vi "data_load_display_trend_fft_mea_coll_v4.vi"() -> ()   [LabVIEW 2020]
uses:
  <vilib>/Analysis/2dsp.llb/Real FFT.vi
  <vilib>/Utility/file.llb/Read Delimited Spreadsheet (DBL).vi
  <vilib>/Utility/file.llb/Read Delimited Spreadsheet (string).vi
  <vilib>/Analysis/NI_AALPro.lvlib
  <vilib>/rvi/Analysis/host/Public/NI_FpgaMspHost.lvlib
  <vilib>/ptbypt/NI_PtbyPt.lvlib
panel:
  out "x-y":dbl
  out "XY Graph 2":T1(graph)
  out "Waveform Graph":dbl[][](graph)
  out "XY Graph":cluster{dbl[], dbl[]}(graph)
  out "magnitude 2":dbl[](array[numeric])
  out "phase 2":dbl[](array[numeric])
  out "signal from each selected frequency":dbl[][](array[numeric])
  out "ploted signal from each selected frequency":dbl[][](graph)
  out "plot restored signal":dbl[](graph)
  out "restored signal":dbl[](array[numeric])
  out "phase":dbl format="%0.2f"
  out "magnitude":dbl format="%0.2f"
  out "magnitude plot":dbl[](graph)
  out "phase plot":dbl[](graph)
  out "magnitudes":dbl[](array[numeric])
  out "phasees":dbl[](array[numeric])
  out "df (Hz)":dbl
  out "size(s)":i32
  out "xf (frequency)":dbl[](array[numeric])
  in  "decimating factor":i32=3
  out "xf (sample Vs frequency )":dbl[][](array[numeric]) format="%#20_5g"
  out "Imaginary values":dbl[](array[numeric])
  out "real  values":dbl[](array[numeric])
  out "real plot":dbl[](graph)
  out "imaginary plot":dbl[](graph)
  out "Time Domain sequence":cluster{i32, dbl, dbl[]}(graph)
  out "Frequency Interval: delta(f)":dbl
  out "Spectrum plot":cluster{i32, dbl, "spectrum out":dbl[]}(graph)
  out "Remove trend":cluster{"all rows":dbl[], dbl[]}(graph)
  out "Time vs Acceleration  find trend graph":T2(graph)
  out "array w/ subset deleted":dbl[][](array[numeric])
  out "first row":string[][](array[string])
  out "time":dbl[](array[numeric])
  out "Acceleration":dbl[](array[numeric])
  out "Time vs Acceleration graph":cluster{"all rows":dbl[], "all rows":dbl[]}(graph)
  out "stripped path":path
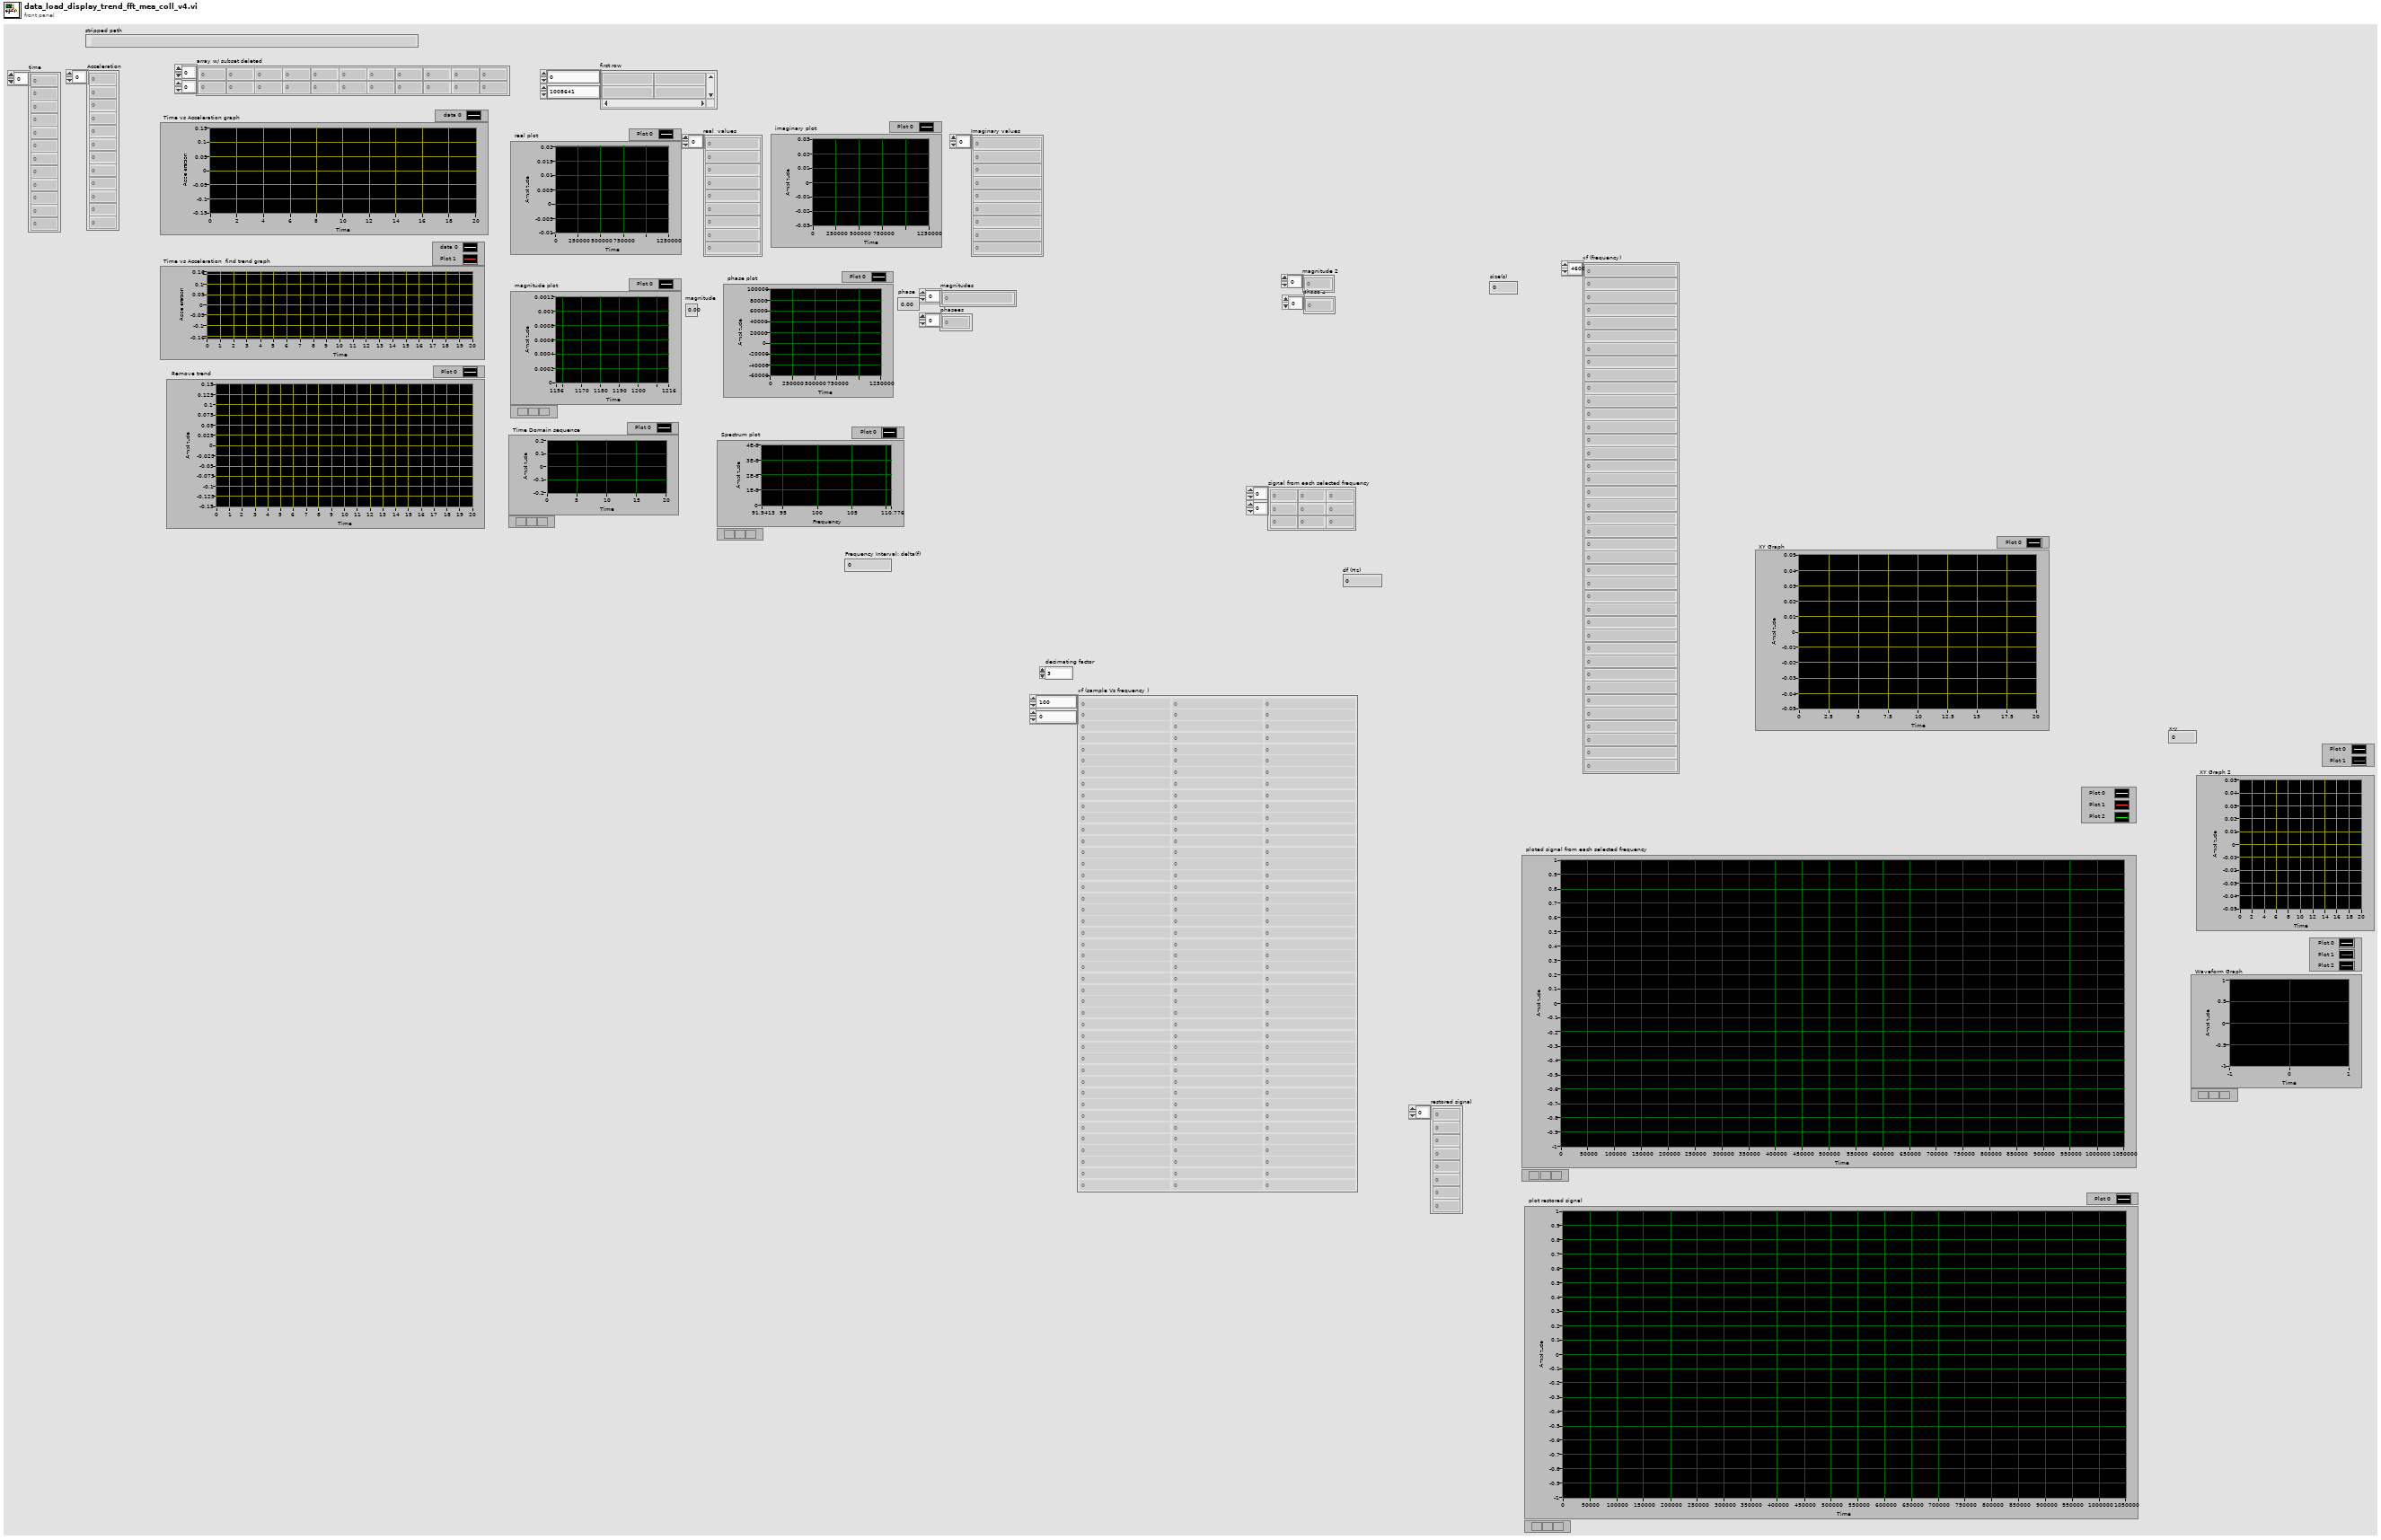
[diagram p1: front panel]
types:
  T1 = cluster{"all rows":dbl[], "Best Linear Fit":dbl[]}[]
  T2 = cluster{"all rows":dbl[], "Best Linear Fit":dbl[]}
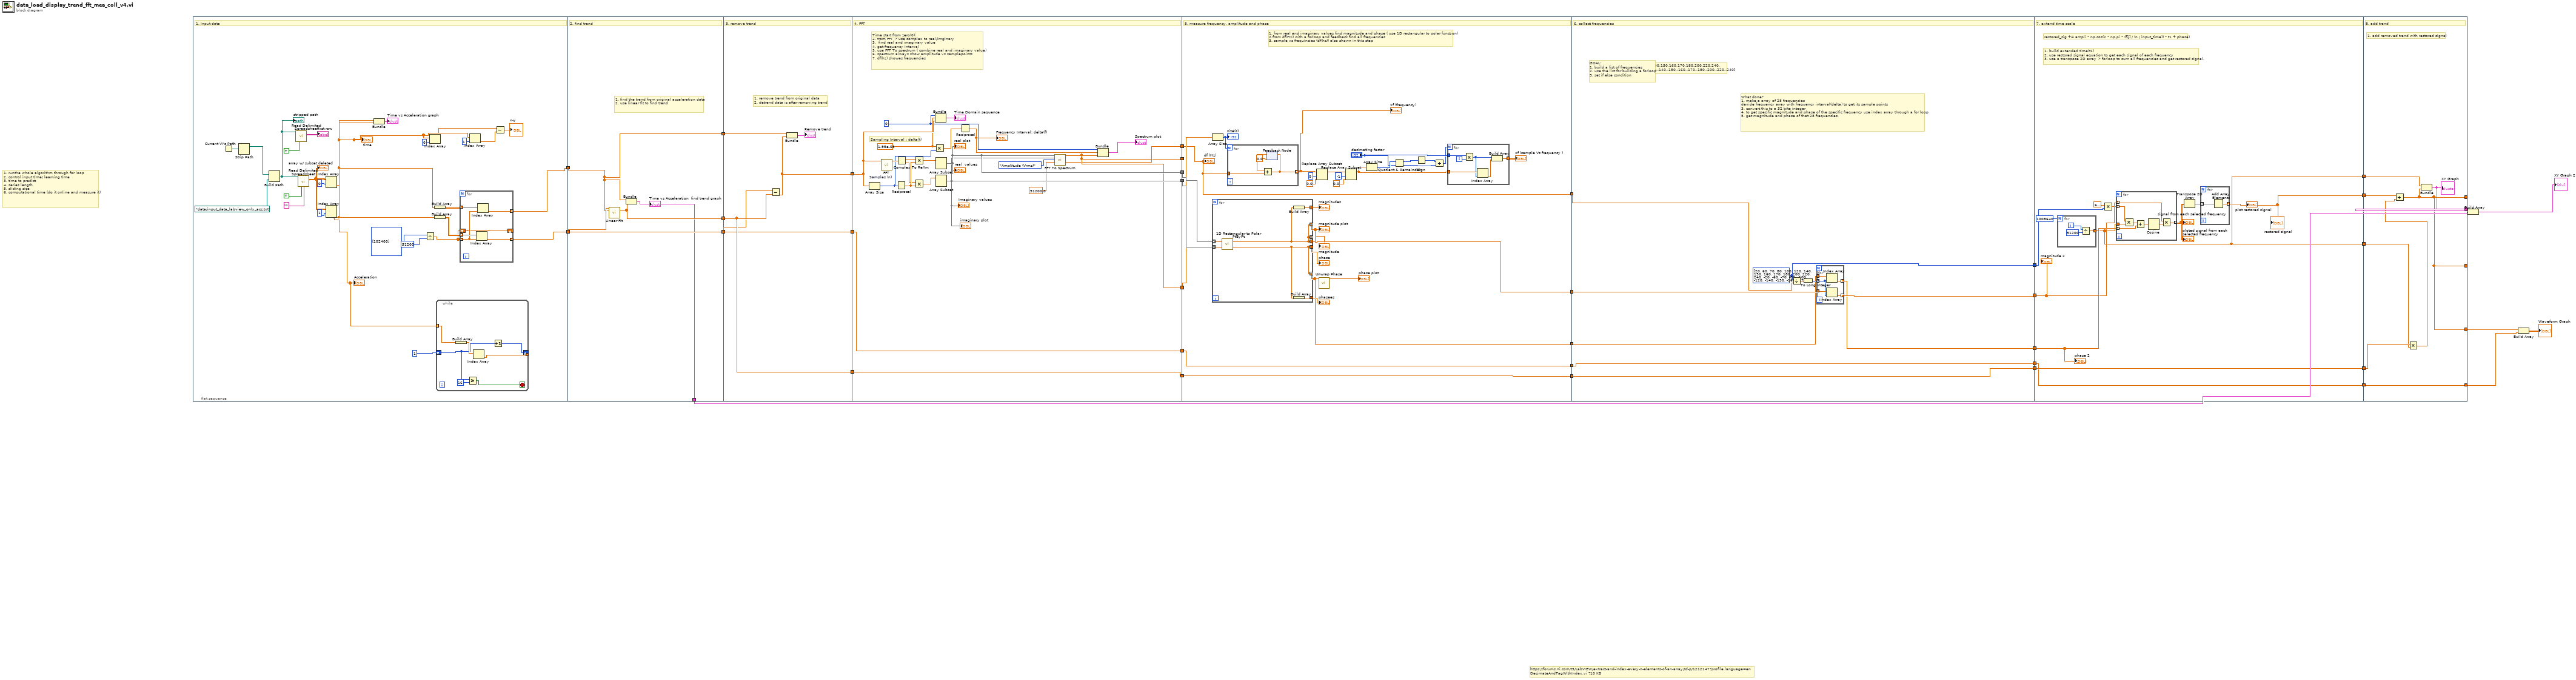
[diagram p0: block diagram]
diagram:
  # "1. runthe whole algorithm through for loop \n2. control input time/ learning time\n3. time to predict\n4. series length\n5. sliding size\n6. computational time (do it online and measure it)"
  # "https://forums.ni.com/t5/LabVIEW/extract-and-index-every-n-elements-of-an-array/td-p/1212147?profile.language=en\nDecimateAndTagWithIndex.vi ?10 KB"
  n1 = flat-sequence {
    tunnel: [w44] -> w36
    tunnel: [w45] -> w35
    tunnel: w36 -> [w79]
    tunnel: [w80] -> w34
    tunnel: [w79] -> w33
    tunnel: [w78] -> w32
    tunnel: w35 -> [w78]
    tunnel: [w77] -> w2
    tunnel: w34 -> [w82]
    tunnel: w33 -> [w81]
    tunnel: w32 -> [w85]
    tunnel: [w84] -> w31
    tunnel: [w82] -> w30
    tunnel: [w81] -> w29
    tunnel: w31 -> [w101]
    tunnel: [w98] -> w28
    tunnel: [w97] -> w27
    tunnel: [w89] -> w26
    tunnel: [w90] -> w25
    tunnel: [w89] -> w24
    tunnel: [w87] -> w23
    tunnel: w30 -> [w87]
    tunnel: w29 -> [w86]
    tunnel: [w86] -> w22
    tunnel: w28 -> [w135]
    tunnel: w27 -> [w134]
    tunnel: w26 -> [_]
    tunnel: w25 -> [w113]
    tunnel: w24 -> [w128]
    tunnel: [w113] -> w21
    tunnel: [w112] -> w20
    tunnel: [w110] -> w19
    tunnel: [w109] -> w18
    tunnel: w23 -> [w109]
    tunnel: w22 -> [w108]
    tunnel: [w108] -> w17
    tunnel: w21 -> [w161]
    tunnel: [w158] -> w16
    tunnel: w20 -> [w157]
    tunnel: w19 -> [w156]
    tunnel: [w155] -> w15
    tunnel: [w154] -> w14
    tunnel: [w153] -> w13
    tunnel: w18 -> [w153]
    tunnel: w17 -> [w152]
    tunnel: [w152] -> w12
    tunnel: w16 -> [w176]
    tunnel: w15 -> [w177]
    tunnel: w14 -> [w172]
    tunnel: [w170] -> w11
    tunnel: [w169] -> w10
    tunnel: w13 -> [w169]
    tunnel: [w168] -> w9
    tunnel: [w168] -> w8
    tunnel: w12 -> [w167]
    tunnel: [w167] -> w7
    tunnel: w11 -> [w199]
    tunnel: w10 -> [w197]
    tunnel: w9 -> [w198]
    tunnel: w8 -> [w196]
    tunnel: [w193] -> _
    tunnel: [w194] -> w5
    tunnel: w7 -> [w194]
    tunnel: [w193] -> _
    tunnel: [w193] -> w6
    tunnel: [w192] -> w3
    frame #0 {
      # "1. Input data"
      n2 = Current VI's Path() -> (path=w55:path)
      n3 = Strip Path(path=w55) -> (stripped path=w54:path)  [unwired: 1 out]
      n4 = Build Path(base path=w54, name or relative path=path "data/input_data_labview_only_acc.txt") -> (appended path=w52:path)
      "stripped path" <- w52
      n5 = call-poly <vilib>:"Read Delimited Spreadsheet.vi"("file path (dialog if empty)"=w52, "transpose? (F)"=TRUE) -> ("all rows"=→"first row":string[][])  [unwired: 8 in, 5 out]
      n6 = call-poly <vilib>:"Read Delimited Spreadsheet.vi"("file path (dialog if empty)"=w52, "transpose? (F)"=TRUE, "delimiter (\\t)"="" ("delimiter (\\t)")) -> ("all rows"=w57:dbl[][])  [unwired: 7 in, 5 out]
      "array w/ subset deleted" <- w57
      n7 = Index Array(array=w57, index (row)=0) -> (element=w42:dbl[])  [unwired: 1 in]
      "time" <- w42
      n8 = Index Array(array=w57, index (row)=1) -> (element=w49:dbl[])  [unwired: 1 in]
      "Acceleration" <- w49
      n9 = Bundle("all rows"=w42, "all rows"=w49) -> (→"Time vs Acceleration graph":cluster{"all rows":dbl[], "all rows":dbl[]})  [unwired: 1 in]
      n10 = Divide(x=i32[] [102400], y=51200) -> (x/y=w43:dbl[])
      n11 = Index Array(array=w42, index=0) -> (element=w39:dbl)
      n12 = Build Array(w42) -> (w50:dbl[][])
      n13 = Build Array(w49) -> (w48:dbl[][])
      n14 = while {
        tunnel: w49 -> [w76] mode=indexing
        tunnel: [w74] -> _ mode=indexing
        shift-right: [w73] -> _
        shift-left: 1 ("index (row)") -> [w72]
        stop <- w70 stop-if-true
        n15 = Build Array(w76) -> (w75:dbl[])
        n16 = Greater Or Equal?(x=w72, y=16) -> (x >= y?=w70:bool)
        n17 = Index Array(array=w75) -> (element=w74:dbl)  [unwired: 1 in]
        n18 = Increment(x=w72) -> (x+1=w73:i32)
      }
      n19 = for {
        tunnel: w50 -> [w69] mode=indexing
        tunnel: w48 -> [w68] mode=indexing
        tunnel: w43 -> [w67] mode=indexing
        tunnel: [w66] -> w45 mode=indexing
        tunnel: [w65] -> w44 mode=indexing
        shift-right: [w64] -> _
        shift-left: w43 -> [w64]
        n20 = Index Array(array=w68, index=w67) -> (element=w65:dbl)
        n21 = Index Array(array=w69, index=w67) -> (element=w66:dbl)
      }
      n22 = Index Array(array=w42, index=1) -> (element=w38:dbl)
      n23 = Subtract(x=w39, y=w38) -> (x-y=→"x-y":dbl)
    }
    frame #1 {
      # "1. find the trend from original acceleration data\n2. use linear fit to find trend"
      # "2. find trend"
      n24 = call <vilib>:"Linear Fit.vi"("Y"=w79, "X"=w78) -> ("Best Linear Fit"=w80:dbl[])  [unwired: 9 in, 4 out]
      n25 = Bundle(w78, "Best Linear Fit"=w80) -> (w77:cluster{dbl[], "Best Linear Fit":dbl[]})  [unwired: 1 in]
      "Time vs Acceleration  find trend graph" <- w77
    }
    frame #2 {
      # "1. remove trend from original data\n2. detrend data is after removing trend"
      # "3. remove trend"
      n26 = Subtract(x=w81, y=w82) -> (x-y=w84:dbl[])
      n27 = Bundle(w85, w84) -> (→"Remove trend":cluster{dbl[], dbl[]})  [unwired: 1 in]
    }
    frame #3 {
      w99 = 1.95e-05
      w95 = 0
      # "1. FFT of detrend data\n2. from FFT > use complex to real/imginary\n3.  find real and imaginary value\n4. get frequency interval\n5. use FFT To spectrum ( combine real and imaginary value)\n6. spectrum always show amplitude vs samplepoints\n7. df(hz) showes frequencies"
      # "Sampling Interval : delta(t)"
      # "Time start from zero(0)"
      # "4. FFT"
      n28 = Array Size "Samples (n)"(array=w101) -> (size(s)=w91:i32)
      n29 = call-poly <vilib>:"FFT.vi"("X"=w101) -> ("FFT {X}"=w93:cdb[])  [unwired: 9 in, 1 out]
      n30 = Reciprocal(x=w91) -> (1/x=w107:dbl)
      n31 = Complex To Re/Im(x + iy=w93) -> (x=w106:dbl[], y=w105:dbl[])
      n32 = Multiply(x=w106, y=w107) -> (x*y=w103:dbl[])
      n33 = Multiply(x=w105, y=w107) -> (x*y=w104:dbl[])
      n34 = Multiply(x=w99, y=w91) -> (x*y=w102:dbl)
      n35 = Bundle(w95, w99, w101) -> (→"Time Domain sequence":cluster{i32, dbl, dbl[]})  [unwired: 1 in]
      n36 = Array Subset(array=w103) -> (w98:dbl[])  [unwired: 2 in]
      "real  values" <- w98
      "real plot" <- w98
      n37 = Array Subset(array=w104) -> (w97:dbl[])  [unwired: 2 in]
      "Imaginary values" <- w97
      "imaginary plot" <- w97
      n38 = Reciprocal(x=w102) -> (1/x=w92:dbl)
      "Frequency Interval: delta(f)" <- w92
      n39 = call <vilib>:"FFT To Spectrum.vi"("real FFT data"=w98, "imaginary FFT data"=w97, "spectrum type"=enum8{"Power (Vrms^2)", "Amplitude (Vrms)"}."Amplitude (Vrms)", "sample rate (S/s)"=51200.0) -> ("spectrum out"=w89:dbl[], "df (Hz)"=w90:dbl)  [unwired: 9 in, 1 out]
      n40 = Bundle(w95, w92, "spectrum out"=w89) -> (→"Spectrum plot":cluster{i32, dbl, "spectrum out":dbl[]})  [unwired: 1 in]
    }
    frame #4 {
      # "1. from real and imaginary values find magnitude and phase ( use 1D rectangular to polar function)\n2.from df(HZ) with a forloop and feedback find all frequencies \n3. sample vs frequincies (df(hz)) also shown in this step"
      # "5. measure frequency, amplitude and phase"
      n41 = Array Size(array=w128) -> (size(s)=w129:i32)
      "size(s)" <- w129
      n42 = for {
        tunnel: w135 -> [w151] mode=indexing
        tunnel: w134 -> [w150] mode=indexing
        tunnel: [w149] -> w133
        tunnel: [w146] -> w111
        tunnel: [w146] -> w112 mode=indexing
        tunnel: [w149] -> w110 mode=indexing
        tunnel: [w148] -> w132
        tunnel: [w147] -> w131
        tunnel: [w146] -> _ mode=indexing
        n43 = call <vilib>:"1D Rectangular to Polar PtByPt.vi"("y"=w150, "x"=w151) -> ("phase"=w149:dbl, "magnitude"=w146:dbl)
        n44 = Build Array(w146) -> (w148:dbl[])
        n45 = Build Array(w149) -> (w147:dbl[])
      }
      "phase" <- w133
      "magnitude" <- w111
      "magnitude plot" <- w112
      "magnitudes" <- w132
      "phasees" <- w131
      n46 = for {
        N: w129 -> [_]
        tunnel: w113 -> [w144]
        tunnel: [w142] -> w114 mode=indexing
        n47 = feedback #1(0.0) -> (w145:dbl)
        n48 = Add(x=w145, y=w144) -> (x+y=w142:dbl)
        n49 = feedback-in #1(w142) -> ()
      }
      "xf (frequency)" <- w114
      n50 = Replace Array Subset(array=w114, new element=0.0 ("new element/subarray"), index=0) -> (w119:dbl[])
      n51 = call <vilib>:"Unwrap Phase.vi"("Phase"=w110) -> ("Unwrapped Phase"=→"phase plot":dbl[])  [unwired: 9 in, 1 out]
      n52 = Replace Array Subset(array=w119, new element=0.0 ("new element/subarray"), index=-1) -> (w116:dbl[])
      n53 = Array Size(array=w116) -> (size(s)=w127:i32)
      n54 = Quotient & Remainder(x=w127, y="decimating factor") -> (x-y*floor(x/y)=w125:i32, floor(x/y)=w124:i32)
      n55 = Sign(1:w125) -> (0:w123:i32)
      n56 = Add(x=w123, y=w124) -> (x+y=w122:i32)
      n57 = for {
        N: w122 -> [_]
        tunnel: w116 -> [w141]
        tunnel: [w138] -> w115 mode=indexing
        tunnel: "decimating factor" -> [w137]
        i -> [w140]
        n58 = Multiply(x=w137, y=w140) -> (x*y=w136:i32)
        n59 = Index Array(array=w141, index=w136) -> (element=w139:dbl)
        n60 = Build Array(w136, w139) -> (w138:dbl[])
      }
      "xf (sample Vs frequency )" <- w115
      "df (Hz)" <- w113
    }
    frame #5 {
      w154 = i32[] [20, 60, 70, 80, 100, 120, 140, 150, 160, 170, 180, 200, 220, 240, -20, -60, -70, -80, -100, -120, -140, -150, -160, -170, -180, -200, -220, -240]
      # "What done?\n1. make a array of 28 frequencies\ndevide frequency array with frequency interval(delta) to get its sample points\n3. convert this to a 32 bite integer\n4. to get specific magnitude and phase of the specific frequency use index array through a for loop\n5. get magnitude and phase of that 28 frequencies."
      # "freq_list = [20,60,70,80,100,120,140,150,160,170,180,200,220,240,\n                -20,-60,-70,-80,-100,-120,-140,-150,-160,-170,-180,-200,-220,-240]"
      # "GOAL:\n1. build a list of frequencies\n2. use the list for building a forloop\n3. set if else condition"
      # "6. collect frequencies"
      n61 = Divide(x=w154, y=w161) -> (x/y=w160:dbl[])
      n62 = To Long Integer(number=w160) -> (32bit integer=w159:i32[])
      n63 = for {
        tunnel: w159 -> [w164] mode=indexing
        tunnel: w157 -> [w166]
        tunnel: [w165] -> w158 mode=indexing
        tunnel: w156 -> [w163]
        tunnel: [w162] -> w155 mode=indexing
        n64 = Index Array(array=w163, index=w164) -> (element=w162:dbl)
        n65 = Index Array(array=w166, index=w164) -> (element=w165:dbl)
      }
    }
    frame #6 {
      # "1. build extended time(t1)\n2. use restored signal equation to get each signal of each frequency\n3. use a transpose 2D array > forloop to sum all frequencies and get restored signal."
      # "restored_sig += ampli * np.cos(2 * np.pi * (f[j] / (n / input_time)) * t1 + phase)"
      # "7. extend time scale"
      n66 = for {
        N: 1008640 -> [_]
        tunnel: [w181] -> w168 mode=indexing
        i -> [w183]
        n67 = Divide(x=w183, y=51200) -> (x/y=w181:dbl)
      }
      n68 = Multiply(x=6.283185307179586, y=w172) -> (x*y=w171:dbl[])
      n69 = for {
        tunnel: w168 -> [w191]
        tunnel: w177 -> [w189] mode=indexing
        tunnel: w176 -> [w188] mode=indexing
        tunnel: [w187] -> w175 mode=indexing
        tunnel: w171 -> [w186] mode=indexing
        n70 = Multiply(x=w186, y=w191) -> (x*y=w190:dbl[])
        n71 = Add(x=w190, y=w189) -> (x+y=w185:dbl[])
        n72 = Cosine(x=w185) -> (cos(x)=w184:dbl[])
        n73 = Multiply(x=w188, y=w184) -> (x*y=w187:dbl[])
      }
      "signal from each selected frequency" <- w175
      "ploted signal from each selected frequency" <- w175
      n74 = Transpose 2D Array(2D array=w175) -> (transposed array=w174:dbl[][])
      n75 = for {
        tunnel: w174 -> [w180] mode=indexing
        tunnel: [w179] -> w170 mode=indexing
        n76 = Add Array Elements(numeric array=w180) -> (sum=w179:dbl)
      }
      "plot restored signal" <- w170
      "restored signal" <- w170
      "magnitude 2" <- w176
      "phase 2" <- w177
    }
    frame #7 {
      # "1. add removed trend with restored signal"
      # "8. add trend"
      n77 = Multiply(x=w197, y=w196) -> (x*y=w195:dbl[])
      n78 = Add(x=w199, y=w195) -> (x+y=w193:dbl[])
      n79 = Bundle(w198, w193) -> (w192:cluster{dbl[], dbl[]})  [unwired: 1 in]
      "XY Graph" <- w192
    }
  }
  n80 = Build Array(w3, w2) -> (→"XY Graph 2":cluster{dbl[], "Best Linear Fit":dbl[]}[])
  n81 = Build Array(w6, w5) -> (→"Waveform Graph":dbl[][])
